vi "Condition Type.vi"(11 "OutOfRange Condition Config in":refnum<class "OutOfRange Condition Config.lvclass">) -> (2 "Condition Type":string)   [LabVIEW 2020, in "VolatusSeqConfig.lvlib" / "OutOfRange Condition Config.lvclass"]
uses:
  OutOfRange Condition Config.lvclass
  OutOfRange Condition Config.lvclass/OutOfRange Condition Config.ctl
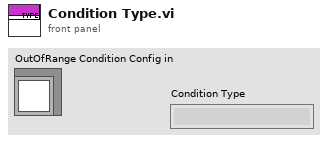
[diagram p1: front panel]
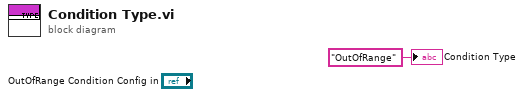
[diagram p0: block diagram]
diagram:
  "Condition Type" <- "OutOfRange" ("Condition Type")
